vi "Move Label.vi"(0 "FSM.Graph In":refnum<class "FSM.Graph.lvclass">, 7 "edgeIndex":i32, 9 "pointIndex":i32) -> (4 "FSM.Graph Out":refnum<class "FSM.Graph.lvclass">)   [LabVIEW 2020, in "FSM.Graph.lvclass"]
uses:
  FSM.Graph.lvclass
  FSM.Graph.lvclass/FSM.Graph.ctl
  FSM.Edge/FSM.Edge.lvclass
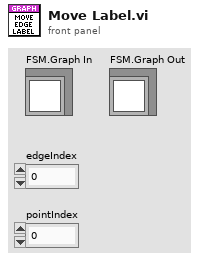
[diagram p1: front panel]
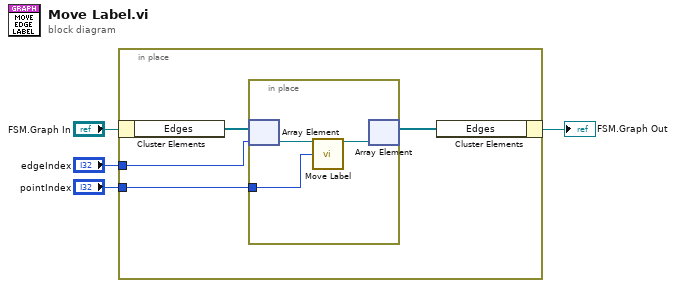
[diagram p0: block diagram]
diagram:
  n1 = in-place {
    in-place-border: "edgeIndex" -> [w8]
    in-place-border: "pointIndex" -> [w5]
    n2 = in-place-cluster #1("FSM.Graph In") -> ("Edges"=w6:refnum<class "FSM.Edge.lvclass">[])
    n3 = in-place {
      in-place-border: w5 -> [w9]
      n4 = in-place-array #2(w6, w8) -> (w11:refnum<class "FSM.Edge.lvclass">)
      n5 = call "Move Label.vi"("FSM.Edge In"=w11, "pointIndex"=w9) -> ("FSM.Edge Out"=w10:refnum<class "FSM.Edge.lvclass">)  [unwired: 13 in]
      n6 = in-place-array #2(w10) -> (w7:refnum<class "FSM.Edge.lvclass">[])  [unwired: 1 out]
    }
    n7 = in-place-cluster #1("Edges"=w7) -> (→"FSM.Graph Out":refnum<class "FSM.Graph.lvclass">)
  }
